vi "Config - OpenConnection.vi"(8 "Fehler (Eingang, kein Fehler)":errorcluster, 10 "Mode":T1(ring), 11 "IP/DNS":string) -> (0 "Fehler (Ausgang)":errorcluster)   [LabVIEW 2016]
uses:
  eGateUtility.dll
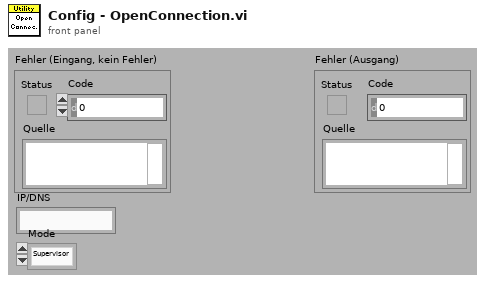
[diagram p1: front panel]
types:
  T1 = enum16{"Supervisor", "Configuration", "Datatransfer"}
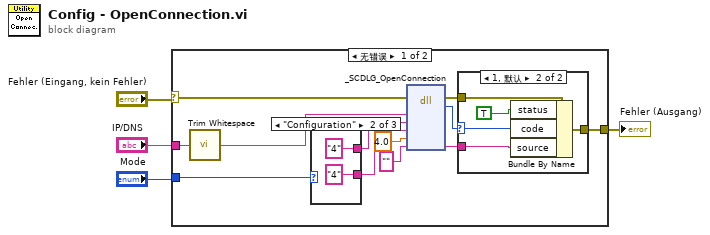
[diagram p0: block diagram]
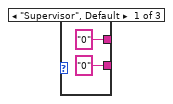
[diagram p3: hidden frame]
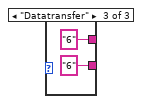
[diagram p4: hidden frame]
diagram:
  n1 = case shown="无错误" "Fehler (Eingang, kein Fehler)" {
    selector: "Fehler (Eingang, kein Fehler)" -> [w14 w29]
    tunnel: [w11 w29] -> w3
    tunnel: "IP/DNS" -> [w6 _]
    tunnel: "Mode" -> [w13 _]
    frame No Error {
      n2 = call <vilib>:"Trim Whitespace.vi"("string"=w6) -> ("trimmed string"=w5:string)  [unwired: 1 in]
      n3 = case shown="\"Configuration\"" w13 {
        tunnel: ["0" ("ErrorString") "4" ("ErrorString") "6" ("ErrorString")] -> w7
        tunnel: ["0" ("ErrorString") "4" ("ErrorString") "6" ("ErrorString")] -> w8
        frame "Supervisor", Default {
        }
        frame "Configuration" {
        }
        frame "Datatransfer" {
        }
      }
      n4 = dll-call lib="eGateUtility.dll" fn="_SCDLG_OpenConnection"(error in=w14, "ServerName"=w5, "UserName"=w7, "Password"=w8, "Timeout"=4.0, "ErrorString"="") -> (error out=w12:errorcluster, "Rückgabetyp"=w10:i32, "ErrorString"=w9:string)  [unwired: 4 in, 3 out]
      n5 = case shown="1, 默认" w10 {
        selector: w10 -> [_ w19]
        tunnel: w12 -> [w17 w22]
        tunnel: [w17 w21] -> w11
        tunnel: w9 -> [_ w20]
        frame 0 {
        }
        frame 1, Default {
          n6 = Bundle By Name(cluster=w22, "status"=TRUE, "code"=w19, "source"=w20) -> (w21:errorcluster)
        }
      }
    }
    frame Error {
    }
  }
  "Fehler (Ausgang)" <- w3
